vi "Ungroup Channels.vi"(8 "error in (no error)":errorcluster {"code" format="%.0x"}, 9 "Ungroup All? (F:False)":bool, 10 "Channel Name (1)":string="1", 11 "VISA resource name":refnum<visa-resource-name>) -> (0 "error out":errorcluster {"code" format="%.0x"}, 3 "VISA resource name out":refnum<visa-resource-name>)   [LabVIEW 2016, in "Agilent N6700 Series.lvlib"]
doc: "Restores a group of channels that have been grouped with <B>Configure Channel Grouping.vi</B> back to an ungrouped state. When ungrouping channels, you must also remove all paralleled connections between the output and sense terminals of that channel.\n\nThis VI deletes any previously saved states. However, for the group changes to take effect, you must also reboot the unit.\n\n<b>Note:</b>\nThis VI does not apply to models N678xA SMU."
uses:
  <instrlib>/Agilent N6700 Series/Agilent N6700 Series.lvlib
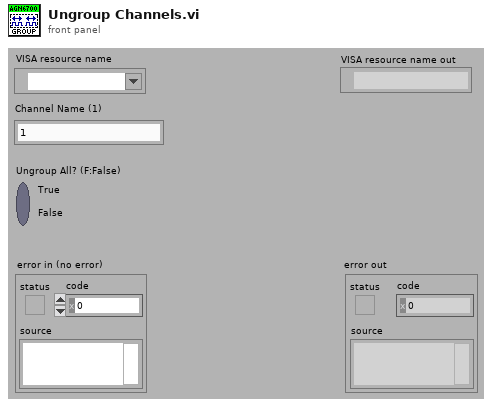
[diagram p1: front panel]
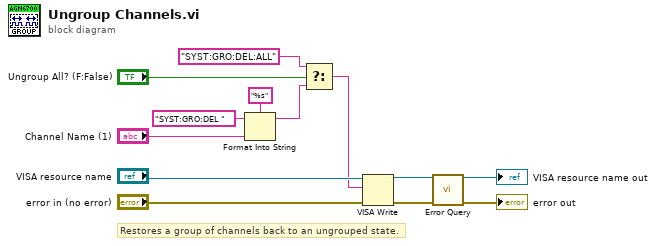
[diagram p0: block diagram]
diagram:
  # "Restores a group of channels back to an ungrouped state."
  n1 = Format Into String(format string="%s", initial string="SYST:GRO:DEL ", "Channel Name (1)") -> (resulting string=w3:string)  [unwired: 1 in, 1 out]
  n2 = Select(t="SYST:GRO:DEL:ALL", s="Ungroup All? (F:False)", f=w3) -> (s? t:f=w1:string)
  n3 = VISA Write(VISA resource name="VISA resource name", write buffer=w1, error in (no error)="error in (no error)") -> (VISA resource name out=w9:refnum<visa-resource-name>, error out=w8:errorcluster)  [unwired: 1 out]
  n4 = call <instrlib>:"Error Query.vi"("VISA resource name"=w9, "error in (no error)"=w8) -> ("VISA resource name out"=→"VISA resource name out":refnum<visa-resource-name>, "error out"=→"error out":errorcluster)  [unwired: 10 in, 2 out]
